vi "IntegrateGyroscopeData.vi"() -> ()   [LabVIEW 2024]
uses:
  <vilib>/Instr/_visa.llb/VISA Configure Serial Port (Instr).vi
panel:
  in  "baud rate":u32=115200
  out "Waveform Chart Outliers Removed":cluster{dbl, dbl, dbl}(graph)
  in  "remove initial offset":bool=TRUE
  out "Relative orientation":T1(graph)
  in  "reset integrator":bool
  out "Yaw angle":dbl format="%#_5g"
  out "Pitch angle":dbl format="%#_5g"
  out "Roll angle":dbl format="%#_5g"
  in  "VISA resource name":refnum<visa-resource-name>="COM8"
  out "Waveform Chart w/ Outliers":sgl[][](graph)
  out "dt (ms)":u32
  out "freq (hz)":dbl
  in  "stop":bool
  # "baud rate must be 9600 > arduino: Serial.begin(9600);"
  # "Select!"
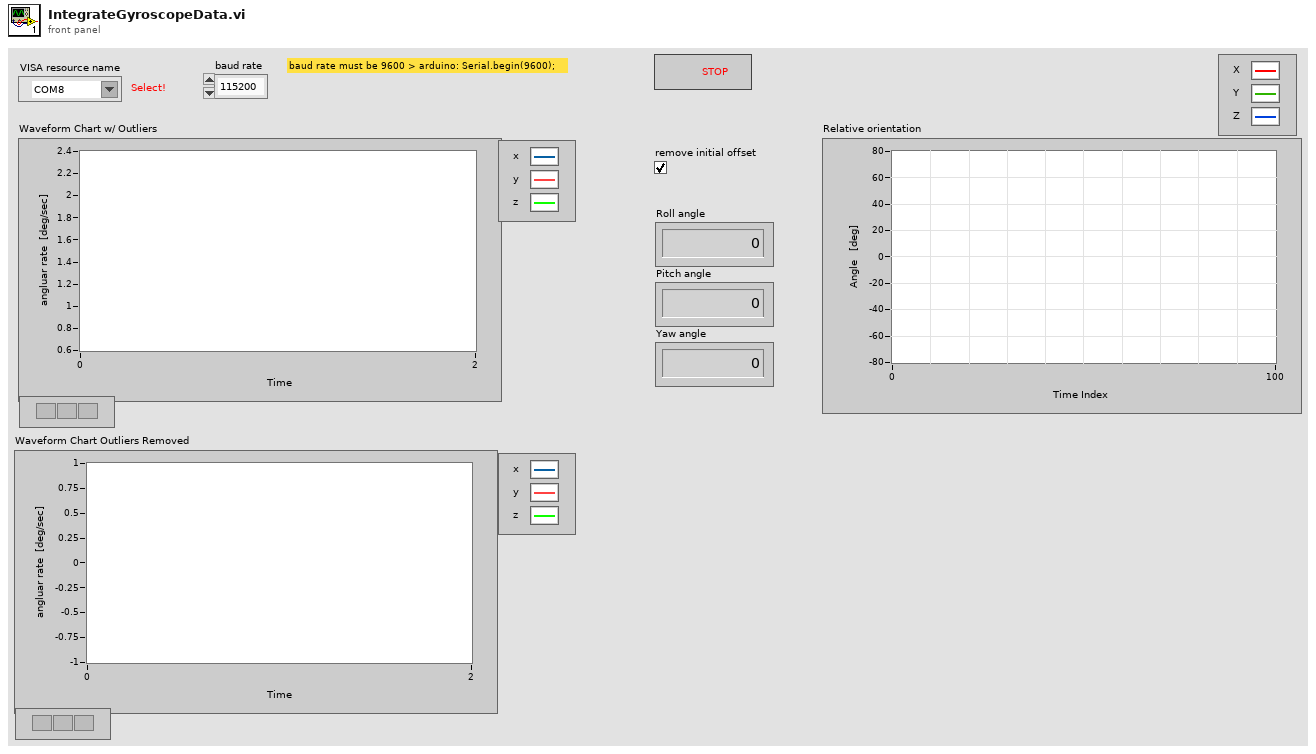
[diagram p1: front panel]
types:
  T1 = cluster{"integral x(t)":dbl, "integral x(t)":dbl, "integral x(t)":dbl}
  T2 = cluster{"median":dbl, "median":dbl, "median":dbl}
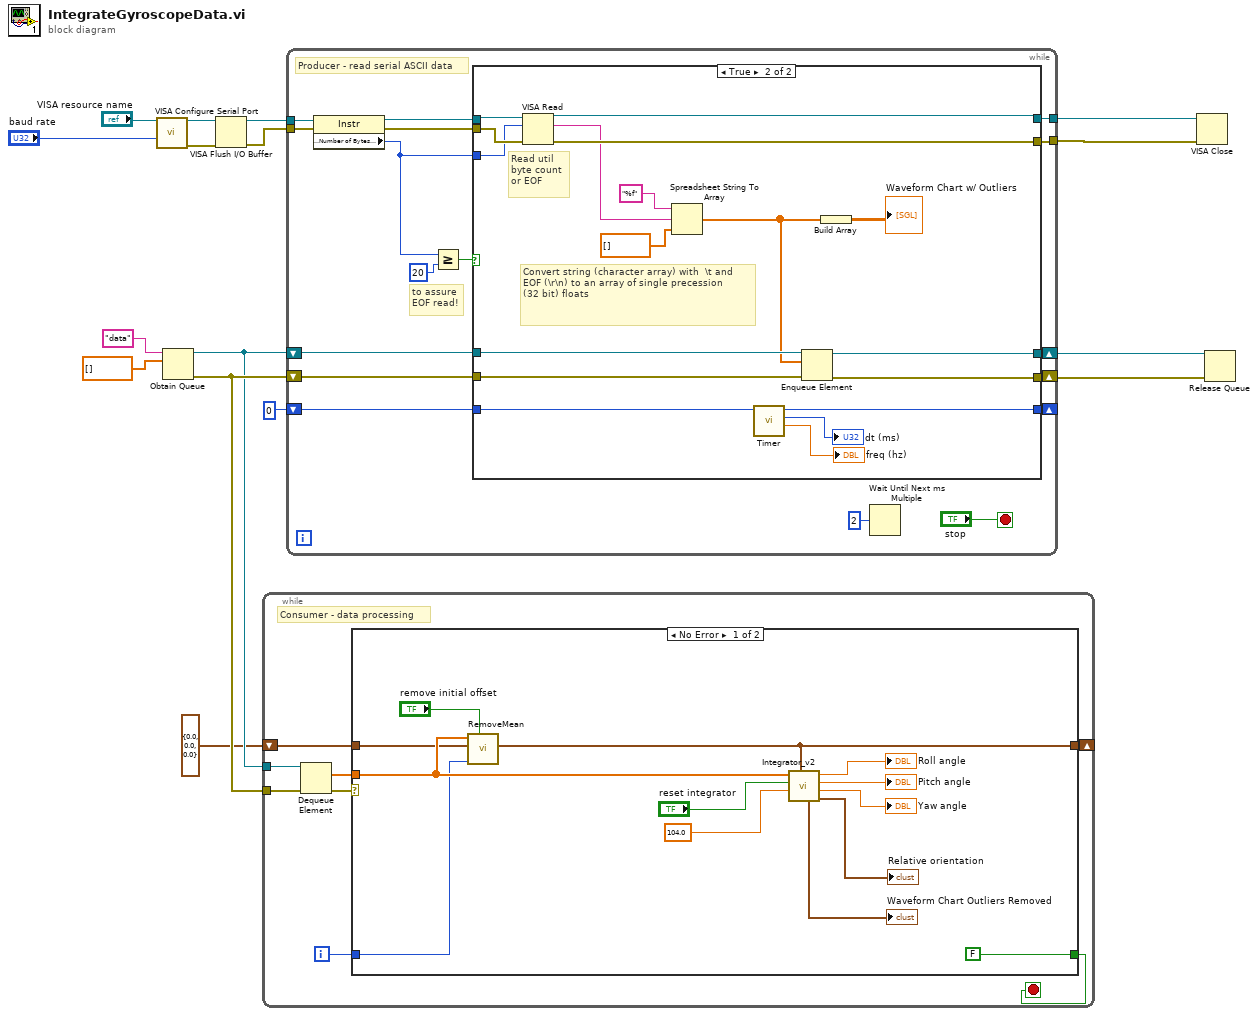
[diagram p0: block diagram]
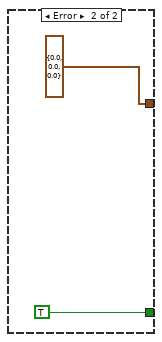
[diagram p2: hidden frame]
diagram:
  n1 = call-poly "VISA Configure Serial Port"("VISA resource name"="VISA resource name", "baud rate (9600)"="baud rate") -> ("VISA resource name out"=w13:refnum<visa-resource-name>, "error out"=w12:errorcluster)  [unwired: 12 in]
  n2 = Obtain Queue(name (unnamed)="data", element data type=sgl[] [] ("array")) -> (queue out=w3:refnum<queue>, error out=w4:errorcluster)  [unwired: 3 in, 1 out]
  n3 = VISA Flush I/O Buffer(VISA resource name=w13, error in (no error)=w12) -> (VISA resource name out=w11:refnum<visa-resource-name>, error out=w10:errorcluster)  [unwired: 1 in]
  n4 = while {
    tunnel: w4 -> [w24]
    tunnel: w3 -> [w23]
    shift-right: [w18] -> _
    shift-left: T2 {"median"=0.0, "median"=0.0, "median"=0.0} ("median_out") -> [w17]
    i -> [w19]
    stop <- w21 stop-if-true
    # "Consumer - data processing"
    n5 = Dequeue Element(queue=w23, error in (no error)=w24) -> (element=w20:sgl[], error out=w22:errorcluster)  [unwired: 1 in, 2 out]
    n6 = case shown="No Error" w22 {
      tunnel: [FALSE TRUE] -> w21
      tunnel: w20 -> [w31 _]
      tunnel: w19 -> [w30 _]
      tunnel: [w29 T2 {"median"=0.0, "median"=0.0, "median"=0.0} ("median_out")] -> w18
      tunnel: w17 -> [w28 _]
      frame No Error {
        n7 = call "RemoveMean.vi"("remove offset"="remove initial offset", "i"=w30, "median_in"=w28, "Gyro data 3DOF"=w31) -> ("median_out"=w29:T2)  [unwired: 7 in]
        n8 = call "Integrator_v2.vi"("median_w"=w29, "fs"=104.0, "Reset integrator"="reset integrator", "Gyro data 3DOF"=w31) -> ("orientation"=→"Relative orientation":cluster{"Roll":dbl, "Pitch":dbl, "Yaw":dbl}, "Yaw angle"=→"Yaw angle":dbl, "Pitch angle"=→"Pitch angle":dbl, "Roll angle"=→"Roll angle":dbl, "offset removed w/ median"=→"Waveform Chart Outliers Removed":cluster{dbl, dbl, dbl})  [unwired: 3 in]
      }
      frame Error {
      }
    }
  }
  n9 = while {
    tunnel: w11 -> [w56]
    tunnel: w10 -> [w55]
    tunnel: [w52] -> w15
    tunnel: [w51] -> w14
    shift-right: [w44] -> _
    shift-left: u32 0 -> [w45]
    shift-right: [w41] -> w6
    shift-left: w3 -> [w43]
    shift-right: [w40] -> w5
    shift-left: w4 -> [w42]
    stop <- "stop" stop-if-true
    # "Producer - read serial ASCII data"
    # "to assure\nEOF read!"
    n10 = property class="Instr"(reference=w56, error in=w55) -> (reference out=w53:refnum<visa-resource-name>, error out=w54:errorcluster, "Serial Settings:Number of Bytes at Serial Port"=w47:u32)
    n11 = Greater Or Equal?(x=w47, y=u32 20) -> (x >= y?=w48:bool)
    n12 = case shown="True" w48 {
      tunnel: w54 -> [w60 w79]
      tunnel: w53 -> [w61 w78]
      tunnel: w47 -> [_ w77]
      tunnel: [w61 w76] -> w52
      tunnel: [w60 w75] -> w51
      tunnel: w45 -> [w59 w74]
      tunnel: [w59 w73] -> w44
      tunnel: w43 -> [w58 w66]
      tunnel: w42 -> [w57 w65]
      tunnel: [w58 w63] -> w41
      tunnel: [w57 w62] -> w40
      frame False {
      }
      frame True {
        # "Convert string (character array) with  \\t and \nEOF (\\r\\n) to an array of single precession \n(32 bit) floats"
        # "Read util\nbyte count\nor EOF"
        n13 = VISA Read(VISA resource name=w78, byte count=w77, error in (no error)=w79) -> (VISA resource name out=w76:refnum<visa-resource-name>, read buffer=w68:string, error out=w75:errorcluster)  [unwired: 1 out]
        n14 = Spreadsheet String To Array(format string="%f", spreadsheet string=w68, array type (2D Dbl)=sgl[] []) -> (array=w64:sgl[])  [unwired: 1 in]
        n15 = call "Timer.vi"("Previous_ms"=w74) -> ("freq (hz)"=→"freq (hz)":dbl, "dt (ms)"=→"dt (ms)":u32, "Next_ms"=w73:u32)  [unwired: 8 in]
        n16 = Enqueue Element(queue=w66, element=w64, error in (no error)=w65) -> (queue out=w63:refnum<queue>, error out=w62:errorcluster)  [unwired: 1 in, 1 out]
        n17 = Build Array(w64) -> (→"Waveform Chart w/ Outliers":sgl[][])
      }
    }
    n18 = Wait Until Next ms Multiple(millisecond multiple=u32 2) -> ()  [unwired: 1 out]
  }
  n19 = VISA Close(VISA resource name=w15, error in (no error)=w14) -> ()  [unwired: 1 out]
  n20 = Release Queue(queue=w6, error in (no error)=w5) -> ()  [unwired: 1 in, 3 out]
